vi "Send Set Controls.vi"(4 "VI Control Values":refnum<class "tBSONDocument.lvclass">, 5 "Ignore Non-existent Controls":bool, 6 "VI Path":string, 7 "Message Priority (Normal)":T1=enum."Normal", 8 "error in (no error)":errorcluster, 9 "Target Name":string, 10 "Project Path":string, 11 "Message Enqueuer":refnum<class "Message Enqueuer.lvclass">) -> (0 "error out":errorcluster, 3 "Message Enqueuer out":refnum<class "Message Enqueuer.lvclass">)   [LabVIEW 2014, in "tWorkerCommandRunner.lvlib" / "Set Controls.lvclass"]
uses:
  Set Controls.lvclass
  <vilib>/ActorFramework/Message Enqueuer/Message Enqueuer.lvclass
  <vilib>/ActorFramework/Message Enqueuer/Message Priority.ctl
  BSON/tBSONDocument/tBSONDocument.lvclass
  Set Controls.lvclass/Set Controls.ctl
  <vilib>/ActorFramework/Message Enqueuer/Message Enqueuer.lvclass/Message Enqueuer.ctl
  <vilib>/ActorFramework/Message Priority Queue/Priority Enqueue.vi
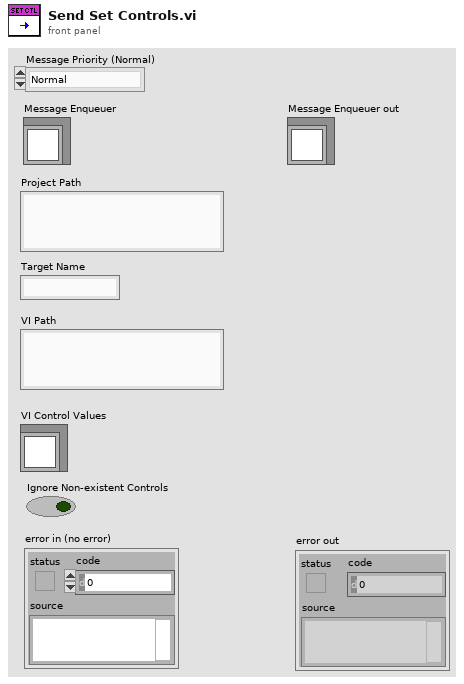
[diagram p1: front panel]
types:
  T1 = typedef "Actor Framework.lvlib/Message Enqueuer.lvclass/Message Priority.ctl" = enum16{"Low", "Normal", "High"}
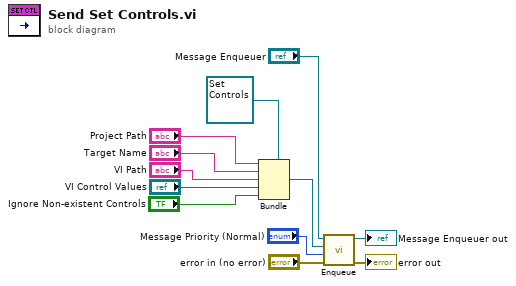
[diagram p0: block diagram]
diagram:
  n1 = Bundle(cluster=refnum<class "Set Controls.lvclass"> refnum ("tWorkerCommandRunner.lvlib:Set Controls.lvclass"), "Project Path", "Target Name", "VI Path", "VI Control Values", "Ignore Non-existent Controls") -> (w9:refnum<class "Set Controls.lvclass">)
  n2 = call <vilib>:"Enqueue.vi"("error in (no error)"="error in (no error)", "Message Priority (Normal)"="Message Priority (Normal)", "Message"=w9, "Message Enqueuer in"="Message Enqueuer") -> ("error out"=→"error out":errorcluster, "Message Enqueuer out"=→"Message Enqueuer out":refnum<class "Message Enqueuer.lvclass">)  [unwired: 6 in]
